vi "BuildArraySampleImage.vi"(11 "chaîne":string) -> (3 "Tableau":string[][](array[string]))   [LabVIEW 2020]
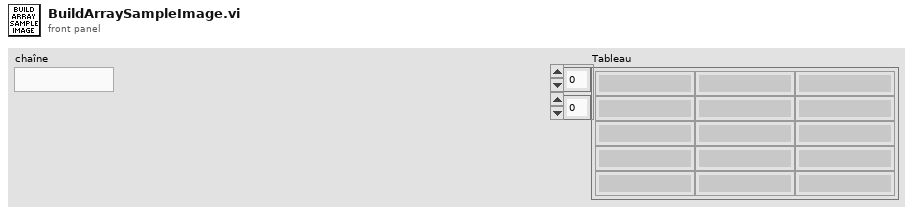
[diagram p1: front panel]
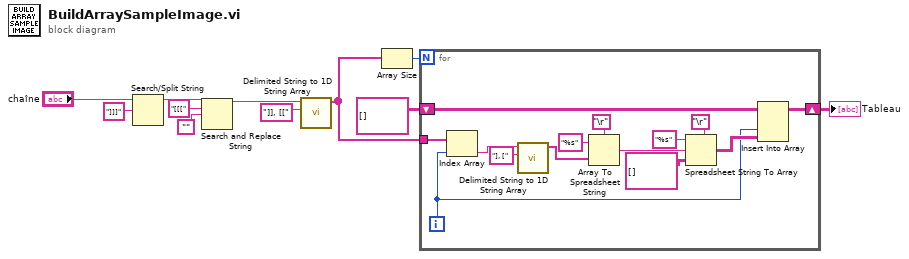
[diagram p0: block diagram]
diagram:
  n1 = Search/Split String(string="chaîne", search string/char (-)="]]]" ("chaîne/car. recherché (-)")) -> (substring before match=w10:string)  [unwired: 1 in, 2 out]
  n2 = Search and Replace String(input string=w10, search string="[[[" ("chaîne recherchée"), replace string="") -> (result string=w6:string)  [unwired: 5 in, 3 out]
  n3 = call <vilib>:"Delimited String to 1D String Array.vi"("delimiter"="]], [[", "delimited string"=w6) -> ("string array"=w3:string[])  [unwired: 9 in]
  n4 = Array Size(array=w3) -> (size(s)=w11:i32)
  n5 = for {
    N: w11 -> [_]
    tunnel: w3 -> [w25]
    shift-right: [w15] -> w1
    shift-left: string[][] [] -> [w16]
    i -> [w12]
    n6 = Index Array(array=w25, index=w12) -> (element=w20:string)
    n7 = call <vilib>:"Delimited String to 1D String Array.vi"("delimiter"="], [", "delimited string"=w20) -> ("string array"=w22:string[])  [unwired: 9 in]
    n8 = Array To Spreadsheet String(delimiter (Tab)="\r", array=w22, 3:"%s" ("chaîne de format")) -> (spreadsheet string=w17:string)
    n9 = Spreadsheet String To Array(delimiter (Tab)="\r", format string="%s" ("chaîne de format"), spreadsheet string=w17, array type (2D Dbl)=string[][] []) -> (array=w14:string[][])
    n10 = Insert Into Array(array=w16, index (col)=w12, new element=w14) -> (w15:string[][])  [unwired: 1 in]
  }
  "Tableau" <- w1
